vi "0.vi"() -> ()   [LabVIEW 2017]
uses:
  <vilib>/Utility/file.llb/Read Delimited Spreadsheet (string).vi
panel:
  out "error out":errorcluster
  out "all rows":string[][](array[string])
  out "prompt (Open existing file)":string
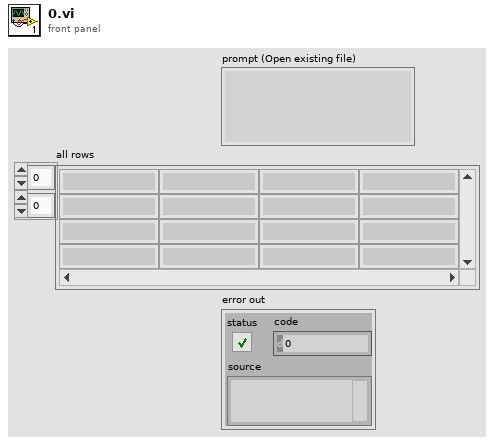
[diagram p1: front panel]
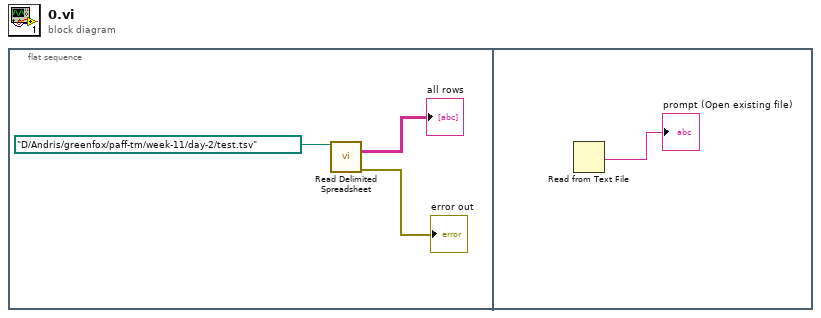
[diagram p0: block diagram]
diagram:
  n1 = flat-sequence {
    frame #0 {
      n2 = call-poly <vilib>:"Read Delimited Spreadsheet.vi"("file path (dialog if empty)"=path "D:/Andris/greenfox/paff-tm/week-11/day-2/test.tsv") -> ("all rows"=→"all rows":string[][], "error out"=→"error out":errorcluster)  [unwired: 9 in, 4 out]
    }
    frame #1 {
      n3 = Read from Text File() -> (text=→"prompt (Open existing file)":string)  [unwired: 4 in, 3 out]
    }
  }
